vi "Enqueue (Array).vi"(4 "timeout in ms (-1)":i32=-1, 6 "Priority Message? Array":bool[](array[boolean]), 8 "error in (no error)":errorcluster, 9 "Message Data Array":variant[](array[variant]), 10 "States":T1[](array[typedef]), 11 "Message Queue":refnum<queue>) -> (0 "error out":errorcluster, 3 "dup Message Queue":refnum<queue>)   [LabVIEW 2019, in "Status.lvlib"]
doc: "For a regular message, enqueue the message. For a priority message, enqueue it at the front of the queue."
uses:
  Status.lvlib
  Queue Type.ctl
  State Name.ctl
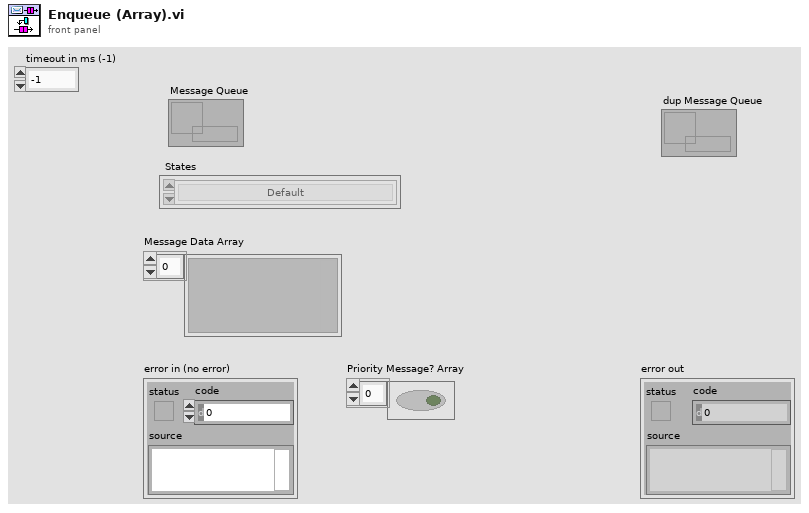
[diagram p1: front panel]
types:
  T1 = typedef "Status.lvlib/State Name.ctl" = enum16{"Initialize", "Update Progress Bar", "Update Status Bar", "Set Cursor Busy", "Unset Cursor Busy", "Error", "Default", "Exit"}
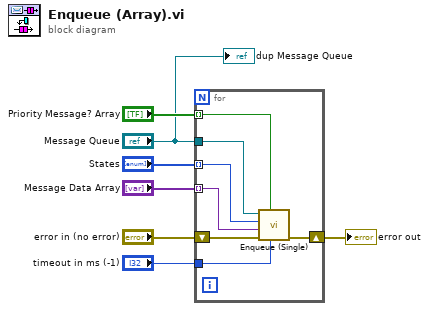
[diagram p0: block diagram]
diagram:
  n1 = for {
    tunnel: "Message Data Array" -> [w13] mode=indexing
    tunnel: "Priority Message? Array" -> [w9] mode=indexing
    tunnel: "Message Queue" -> [w11]
    shift-right: [w10] -> w4
    shift-left: "error in (no error)" -> [w14]
    tunnel: "States" -> [w12] mode=indexing
    tunnel: "timeout in ms (-1)" -> [w8]
    n2 = call "Enqueue (Single).vi"("timeout in ms (-1)"=w8, "Priority Message? Array"=w9, "error in (no error)"=w14, "Message Data Array"=w13, "States"=w12, "Message Queue"=w11) -> ("error out"=w10:errorcluster)  [unwired: 4 in, 1 out]
  }
  "error out" <- w4
  "dup Message Queue" <- "Message Queue"
